vi "OpenPrefdialog.vi"(8 "error in (no error)":errorcluster, 9 "PluginIniFilePath":path, 10 "Class Path":path) -> (0 "error out":errorcluster)   [LabVIEW 2018, in "SensorPlugins.lvlib" / "SensorBase.lvclass"]
uses:
  SensorBase.lvclass
  C:/Program Files/National Instruments/LabVIEW 2018/user.lib/NIST/BaseClasses/BasePlugin_class/BasePlugin.lvclass
  <userlib>/NIST/BaseClasses/BasePlugin_class/BasePlugin.lvclass/BasePlugin.ctl
  <userlib>/NIST/BaseClasses/BasePlugin_class/Accessors/Write PluginIniFilePath.vi
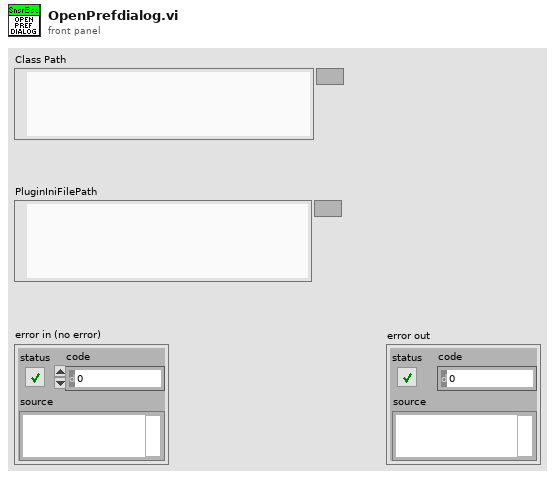
[diagram p1: front panel]
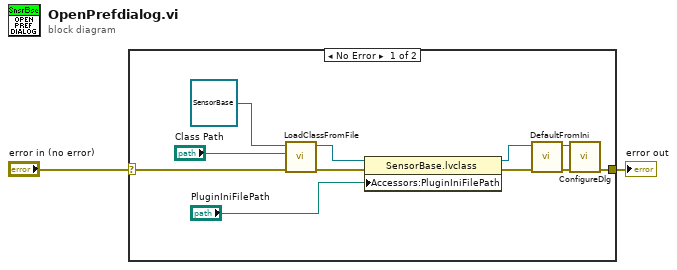
[diagram p0: block diagram]
diagram:
  n1 = case shown="No Error" "error in (no error)" {
    selector: "error in (no error)" -> [w10 w14]
    tunnel: [w4 w14] -> w1
    frame No Error {
      n2 = call-dynamic "LoadClassFromFile.vi"("error in (no error)"=w10, "class path"="Class Path", "reference in"=refnum<class "SensorBase.lvclass"> refnum ("SensorPlugins.lvlib:SensorBase.lvclass")) -> ("error out"=w12:errorcluster, "reference out"=w13:refnum<class "SensorBase.lvclass">)  [unwired: 7 in]
      n3 = property class="SensorBase.lvclass"(reference=w13, error in=w12, "Accessors:PluginIniFilePath"="PluginIniFilePath") -> (reference out=w8:refnum<class "SensorBase.lvclass">, error out=w11:errorcluster)
      n4 = call-dynamic "DefaultFromIni.vi"("error in (no error)"=w11, "SensorBase in"=w8) -> ("error out"=w9:errorcluster, "SensorBase out"=w3:refnum<class "SensorBase.lvclass">)  [unwired: 8 in]
      n5 = call-dynamic "ConfigureDlg.vi"("error in (no error)"=w9, "PmuBase in"=w3) -> ("error out"=w4:errorcluster)  [unwired: 7 in, 2 out]
    }
    frame Error {
    }
  }
  "error out" <- w1
